vi "CA.vi"(0 "States":refnum<vi>, 1 "AlgStates":refnum<vi>, 2 "Processes":refnum<vi>, 3 "INP":refnum<vi>, 4 "PORTS":refnum<vi>) -> ()   [LabVIEW 2010]
uses:
  lib/Ports.lvclass
panel:
  in  "OUTP":refnum<vi>
  out "Value":T1
  out "Состояни процессов":string[][](table)
  in  "OUT Ports Array":cluster{"String":string, "Array 2":bool[]}[](array[cluster])
  in  "INP Ports Array":cluster{"String":string, "Array 2":bool[]}[](array[cluster])
  in  "Значения выходных глобальных переменных":string[][](table)
  in  "Значения входных глобальных переменных":string[][](table)
  out "Выходные сообщения":string[][](table)
  # "Алгоритм управления"
  # "Значения входных портов"
  # "Значения выходных портов"
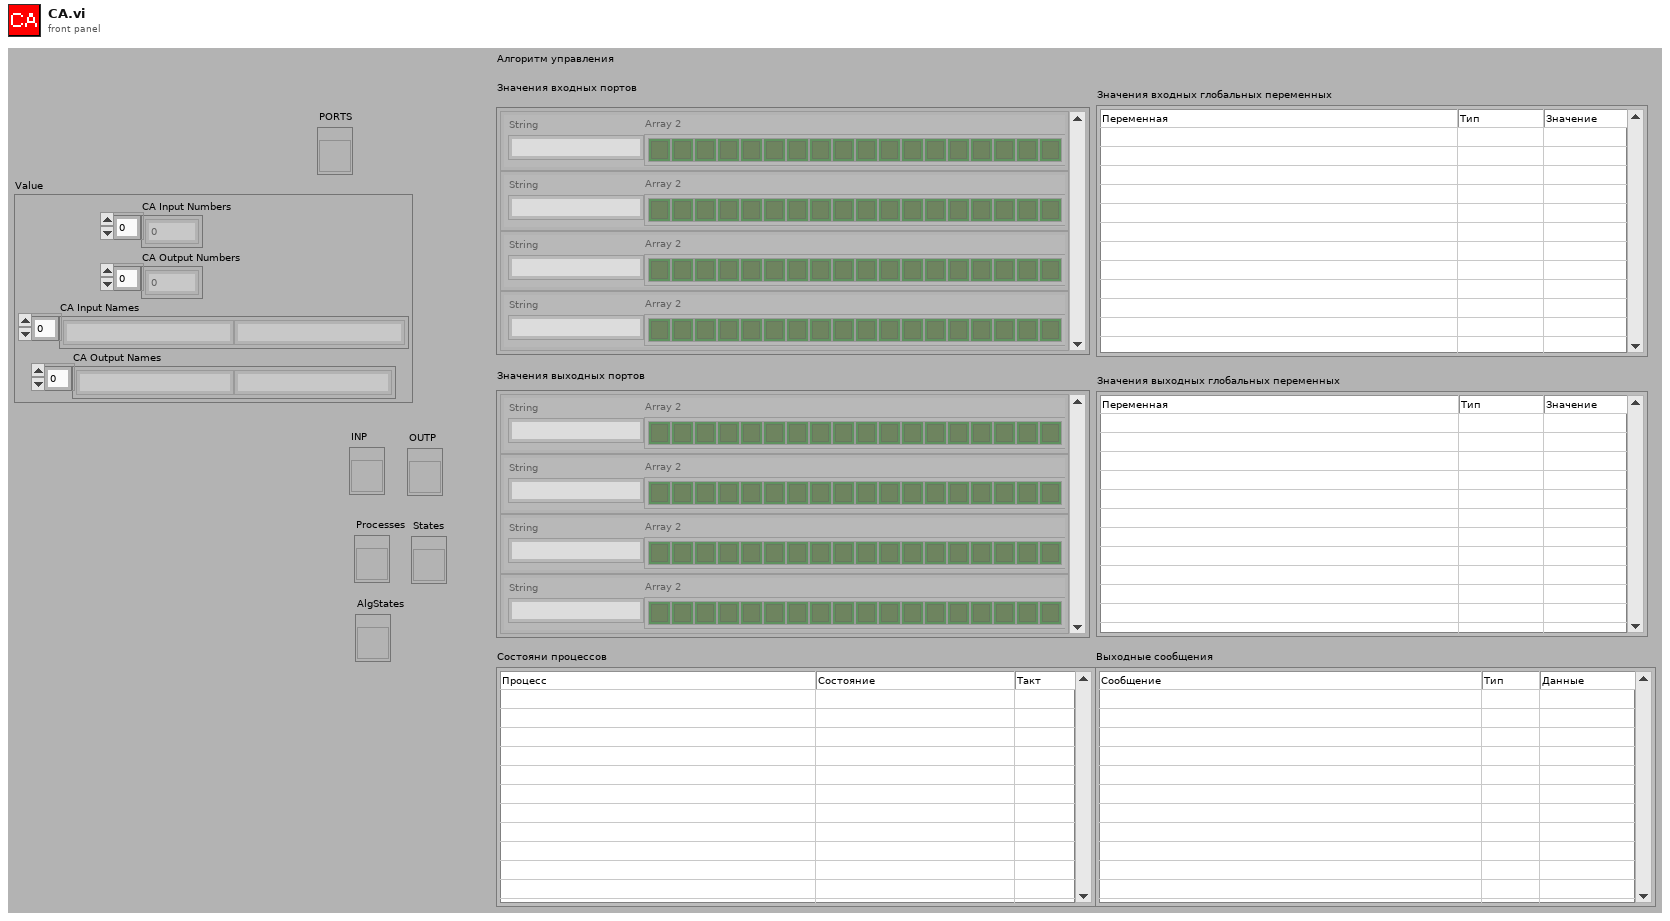
[diagram p1: front panel]
types:
  T1 = cluster{"CA Input Numbers":i32[], "CA Output Numbers ":i32[], "CA Input Names":string[], "CA Output Names ":string[]}
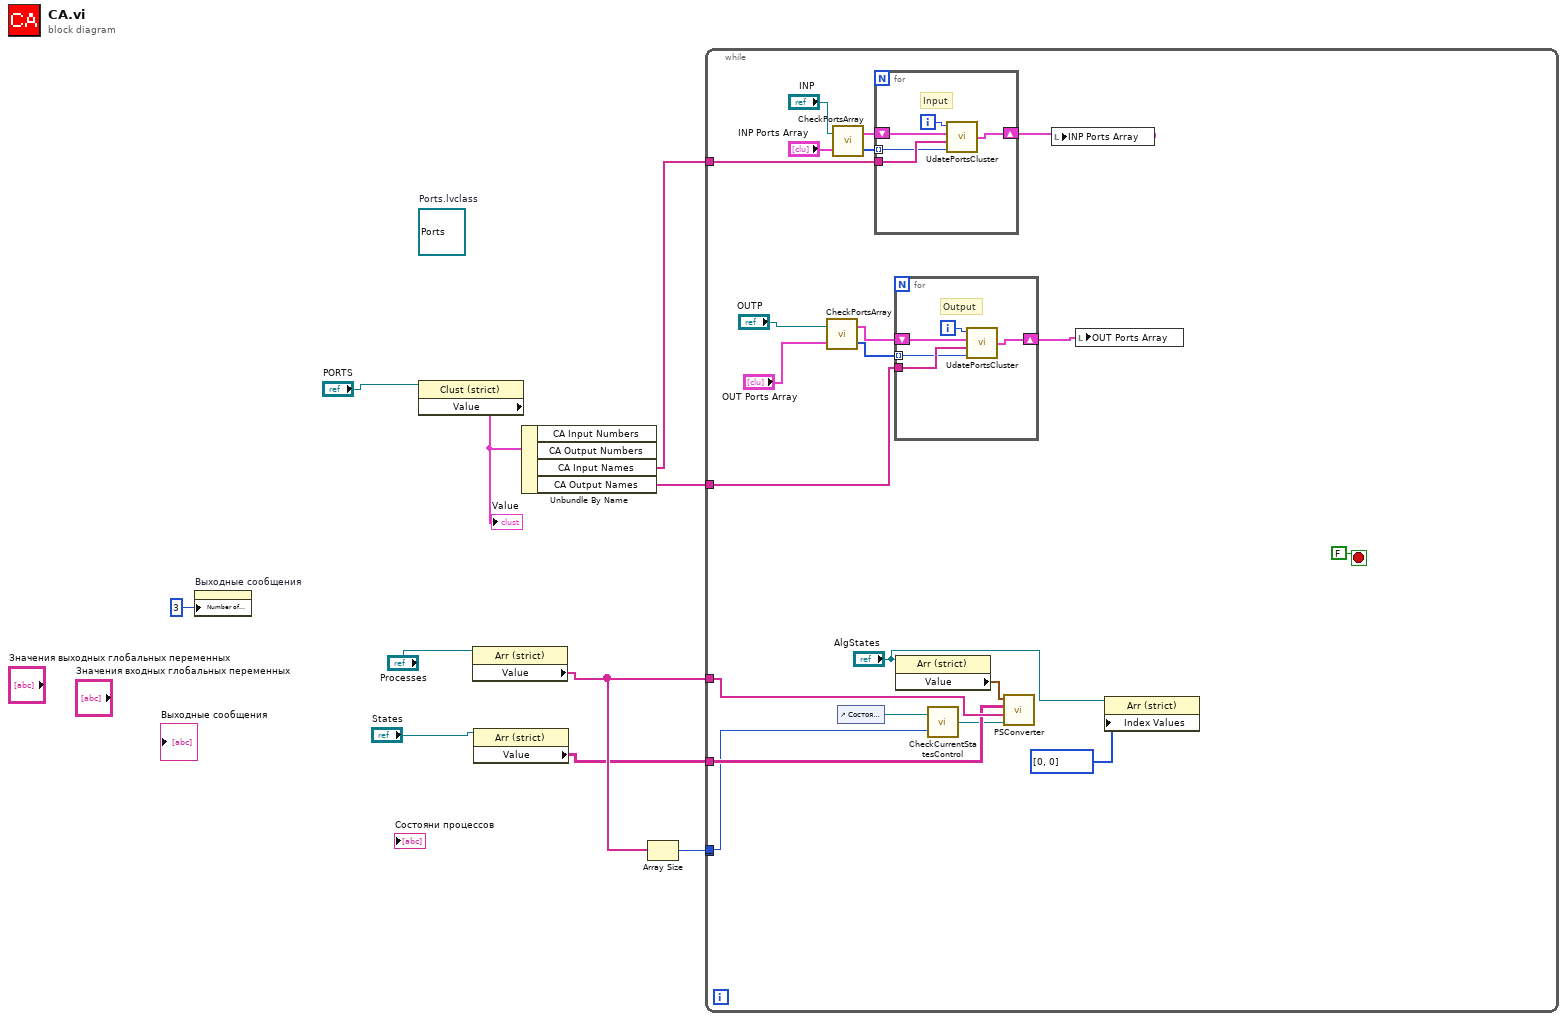
[diagram p0: block diagram]
diagram:
  (unwired) refnum<class "Ports.lvclass"> refnum  # Ports.lvclass
  n1 = property on="Выходные сообщения" class="Tbl (strict)"("Number of Columns"=u32 3 ("Number of Rows")) -> ()  [unwired: 2 in, 2 out]
  n2 = property class="Clust (strict)"(reference="PORTS") -> ("Value"=w8:T1)  [unwired: 1 in, 2 out]
  "Value" <- w8
  n3 = property class="Arr (strict)"(reference="Processes") -> ("Value"=w3:string[])  [unwired: 1 in, 2 out]
  n4 = property class="Arr (strict)"(reference="States") -> ("Value"=w1:string[][])  [unwired: 1 in, 2 out]
  n5 = Unbundle By Name(w8) -> ("CA Input Names"=w7:string[], "CA Output Names"=w6:string[])  [unwired: 2 out]
  n6 = Array Size(array=w3) -> (size(s)=w2:i32)
  n7 = while {
    tunnel: w7 -> [w29]
    tunnel: w6 -> [w21]
    tunnel: w3 -> [w17]
    tunnel: w1 -> [w16]
    tunnel: [w15] -> _
    tunnel: w2 -> [w15]
    stop <- FALSE ("stop") stop-if-true
    n8 = call "CheckPortsArray.vi"("INP Ports Array 2"="OUT Ports Array", "INP"="OUTP") -> ("Value"=w20:i8[], "INP Ports Array"=w22:cluster{"String":string, "Array 2":bool[]}[])
    n9 = call "CheckPortsArray.vi"("INP Ports Array 2"="INP Ports Array", "INP"="INP") -> ("Value"=w28:i8[], "INP Ports Array"=w26:cluster{"String":string, "Array 2":bool[]}[])
    n10 = control-ref of="Состояни процессов"() -> (w14:refnum<vi>)
    n11 = for {
      tunnel: w28 -> [w40] mode=indexing
      tunnel: w29 -> [w41]
      shift-right: [w37] -> w23
      shift-left: w26 -> [w38]
      i -> [w39]
      # "Input"
      n12 = call "UdatePortsCluster.vi"("Numeric 2"=w40, "Input Names"=w41, "Ports Array"=w38, "index"=w39) -> ("INP Ports Array 2"=w37:cluster{"String":string, "Array 2":bool[]}[])
    }
    n13 = for {
      tunnel: w20 -> [w35] mode=indexing
      tunnel: w21 -> [w36]
      shift-right: [w32] -> w19
      shift-left: w22 -> [w33]
      i -> [w34]
      # "Output"
      n14 = call "UdatePortsCluster.vi"("Numeric 2"=w35, "Input Names"=w36, "Ports Array"=w33, "index"=w34) -> ("INP Ports Array 2"=w32:cluster{"String":string, "Array 2":bool[]}[])
    }
    n15 = property class="Arr (strict)"(reference="AlgStates") -> ("Value"=w18:cluster{"TimeInState":u16, "cur_state":i8}[])  [unwired: 1 in, 2 out]
    n16 = call "CheckCurrentStatesControl.vi"("Processes"=w15, "Inp reference"=w14) -> ("Out Refnum"=w13:refnum<vi>)
    n17 = call "PSConverter.vi"("Tbl Refnum"=w13, "PROC"=w17, "STATES"=w16, "Input claster"=w18) -> ()  [unwired: 1 out]
    n18 = local write "INP Ports Array"(w23) -> ()
    n19 = local write "OUT Ports Array"(w19) -> ()
    n20 = property class="Arr (strict)"(reference="AlgStates", "Index Values"=u32[] [0, 0]) -> ()  [unwired: 1 in, 2 out]
  }
